vi "int2.vi"() -> ()   [LabVIEW 2017]
uses:
  <vilib>/picture/3D Picture Control/NI_3D Picture Control.lvlib
panel:
  out "3D Picture":refnum<vi>(3d-picture)
  in  "Stop Button":bool
  in  "Objetos":path
  in  "Mundo":path
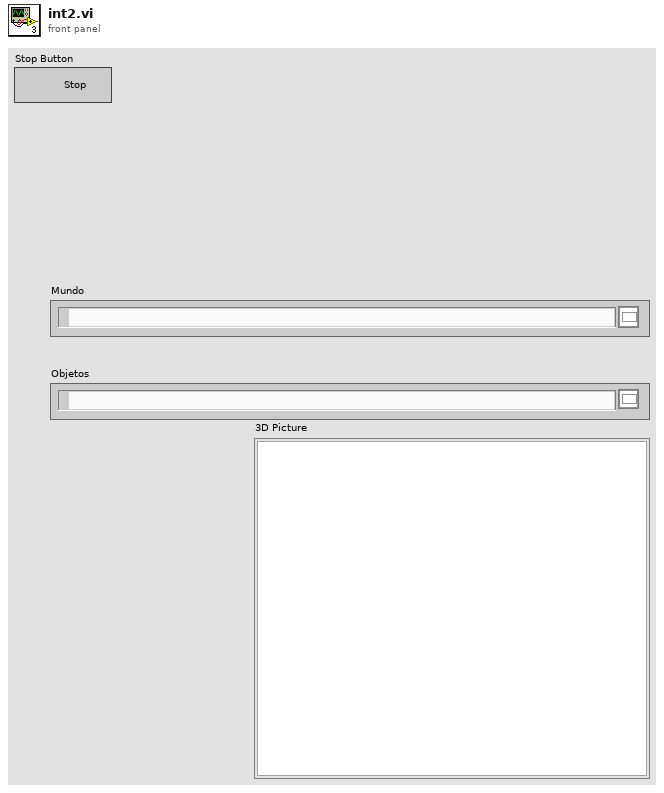
[diagram p1: front panel]
types:
  T1 = enum16{"open", "replace", "create", "open or create", "replace or create", "replace or create with confirmation"}
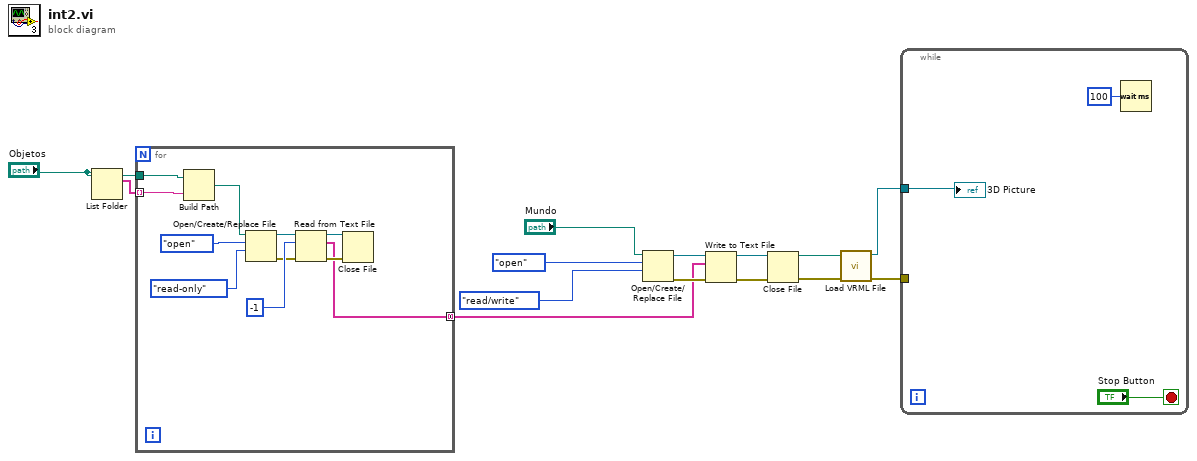
[diagram p0: block diagram]
diagram:
  n1 = List Folder(path="Objetos") -> (filenames=w7:string[])  [unwired: 3 in, 3 out]
  n2 = for {
    tunnel: w7 -> [w25] mode=indexing
    tunnel: "Objetos" -> [w24]
    tunnel: [w15] -> w1 mode=concatenating
    n3 = Build Path(base path=w24, name or relative path=w25) -> (appended path=w23:path)
    n4 = Open/Create/Replace File(file path (use dialog)=w23, operation (0:open)=T1."open", access (0:read/write)=enum16{"read/write", "read-only", "write-only"}."read-only") -> (refnum out=w20:refnum<file>, error out=w18:errorcluster)  [unwired: 3 in, 1 out]
    n5 = Read from Text File(file (use dialog)=w20, count=-1, error in=w18) -> (refnum out=w16:refnum<file>, text=w15:string[], error out=w17:errorcluster)  [unwired: 1 in, 1 out]
    n6 = Close File(refnum=w16, error in=w17) -> ()  [unwired: 2 out]
  }
  n7 = Open/Create/Replace File(file path (use dialog)="Mundo", operation (0:open)=T1."open", access (0:read/write)=enum16{"read/write", "read-only", "write-only"}."read/write") -> (refnum out=w11:refnum<file>, error out=w10:errorcluster)  [unwired: 3 in, 1 out]
  n8 = Write to Text File(file (use dialog)=w11, text=w1, error in=w10) -> (refnum out=w8:refnum<file>, error out=w9:errorcluster)  [unwired: 1 in, 1 out]
  n9 = Close File(refnum=w8, error in=w9) -> (path=w5:path, error out=w4:errorcluster)
  n10 = call <vilib>:"Load VRML File.vi"("error in"=w4, "Path"=w5) -> ("error out"=w2:errorcluster, "Scene:Read Scene File"=w3:refnum<vi>)  [unwired: 8 in]
  n11 = while {
    tunnel: w3 -> [w26]
    tunnel: w2 -> [_]
    stop <- "Stop Button" stop-if-true
    n12 = Wait (ms)(milliseconds to wait=u32 100) -> ()  [unwired: 1 out]
    "3D Picture" <- w26
  }
